vi "Append Inspection Waypoint.vi"(0 "Waypoint Array In":T1[](array[typedef]), 5 "Lat":sgl, 7 "Lon":sgl, 9 "Altitude (m)":sgl, 11 "Error In":errorcluster, 12 "Inspection altitude (m)":sgl=10.0, 13 "Capture Photo":bool) -> (4 "appended array":T1[](array[typedef]), 15 "Error Out":errorcluster)   [LabVIEW 2014]
uses:
  Controls/Mission Planning Controls/MAVLINK Mission Item.ctl
  Controls/MAVLINK Mav Frame.ctl
  Commands/Mission Planning/MISSION_ITEM SubVI/MISSION_ITEM Loiter (Time).vi
  Commands/Mission Planning/MISSION_ITEM SubVI/MISSION_ITEM Condition YAW.vi
  Commands/Mission Planning/MISSION_ITEM SubVI/MISSION_ITEM Take Photo.vi
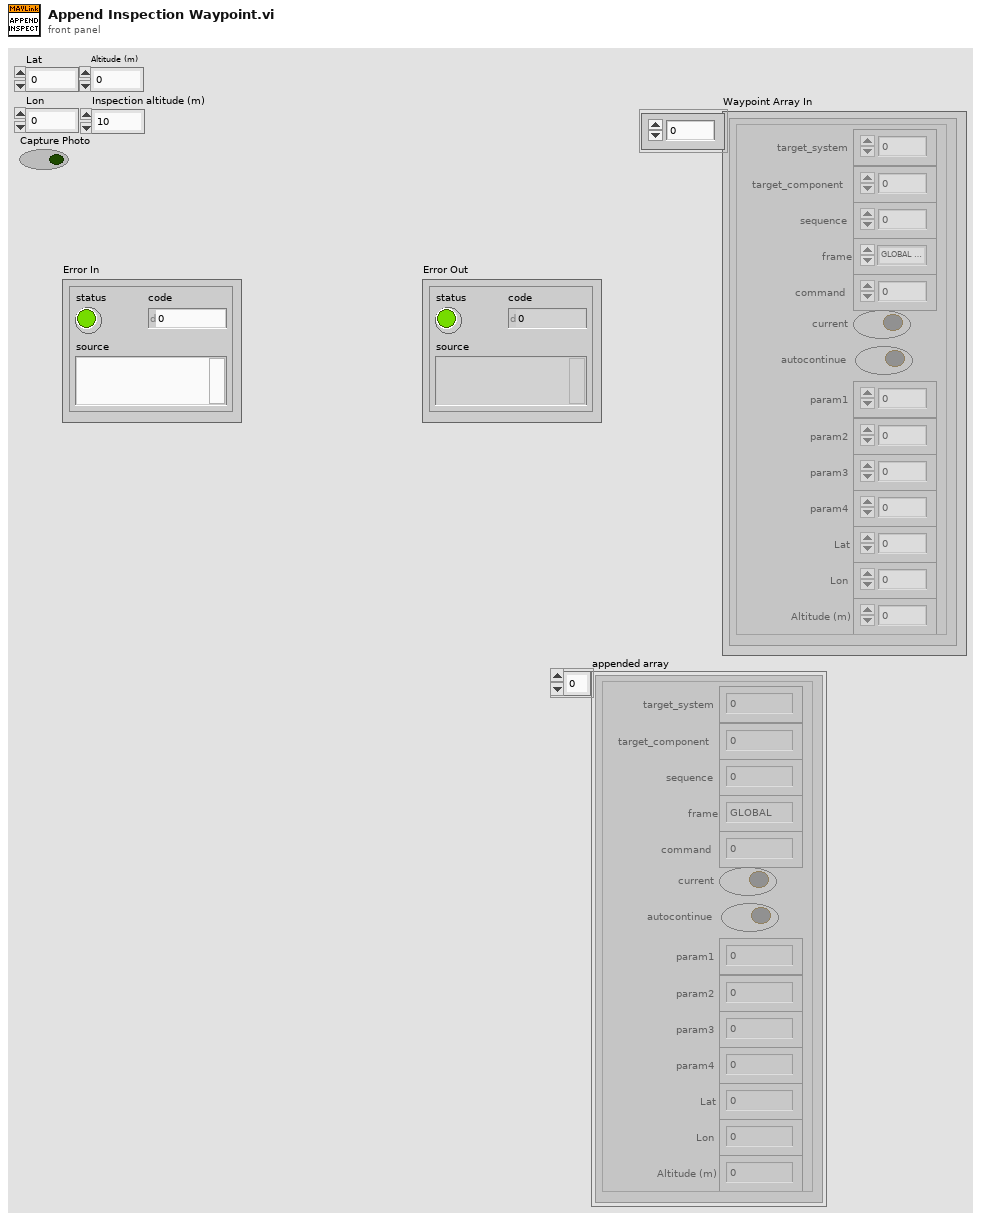
[diagram p1: front panel]
types:
  T1 = typedef "MAVLINK Mission Item.ctl" = cluster{"target_system":u8, "target_component":u8, "sequence":u16, "frame":T2, "command":u16, "current":bool, "autocontinue":bool, "param1":sgl, "param2":sgl, "param3":sgl, "param4":sgl, "Lat":sgl, "Lon":sgl, "Altitude (m)":sgl}
  T2 = typedef "MAVLINK Mav Frame.ctl" = enum8{"GLOBAL", "LOCAL NED", "MISSION", "GLOBAL RELATIVE ALT", "LOCAL ENU", "GLOBAL INT", "GLOBAL RELATIVE ALT INT", "LOCAL OFFSET NED", "BODY NED", "BODY OFFSET NED", "GLOBAL TERRAIN ALT", "GLOBAL TERRAIN ALT INT"}
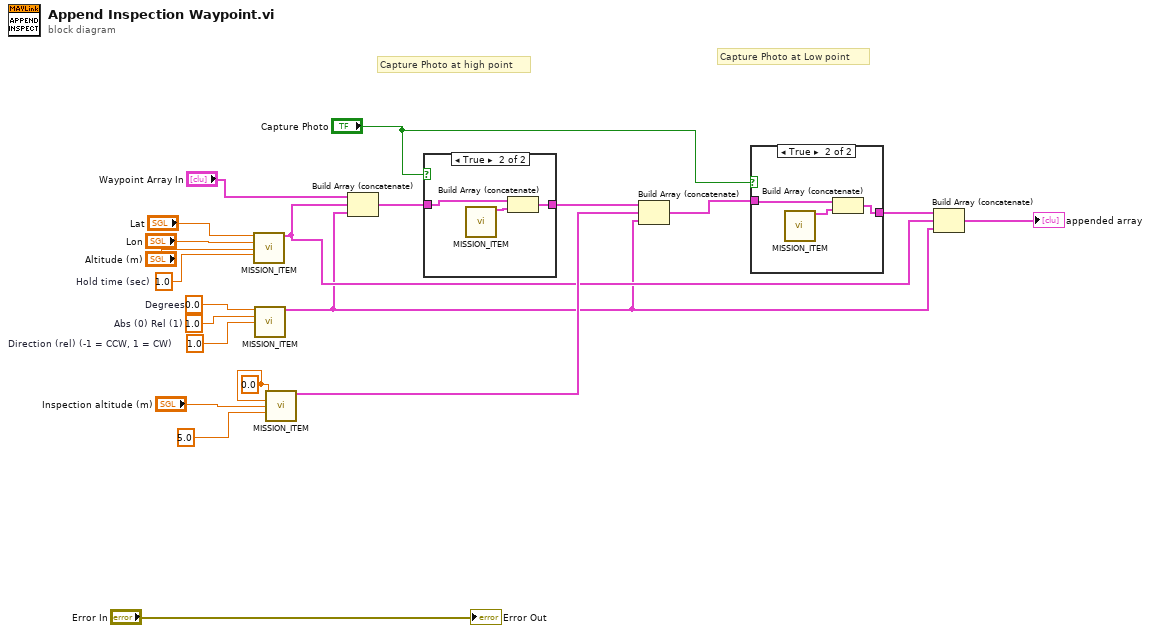
[diagram p0: block diagram]
diagram:
  w11 = sgl 1.0  # Direction (rel) (-1 = CCW, 1 = CW)
  w12 = sgl 1.0  # Abs (0) Rel (1)
  w13 = sgl 0.0  # Degrees
  w15 = sgl 0.0 ("Lat")
  w18 = sgl 1.0  # Hold time (sec)
  # "Capture Photo at Low point"
  # "Capture Photo at high point"
  n1 = call-poly "MISSION_ITEM.vi"("Lat"="Lat", "Lon"="Lon", "Altitude (m)"="Altitude (m)", "Loiter time (sec)"=w18) -> ("Mission Item"=w3:T1)  [unwired: 11 in]
  n2 = call-poly "MISSION_ITEM.vi"("Degrees"=w13, "Abs (0) Rel (1)"=w12, "Direction (rel) (-1 = CCW, 1 = CW)"=w11) -> ("Mission Item"=w2:T1)  [unwired: 12 in]
  n3 = call-poly "MISSION_ITEM.vi"("Lat"=w15, "Lon"=w15, "Altitude (m)"="Inspection altitude (m)", "Loiter time (sec)"=sgl 5.0) -> ("Mission Item"=w7:T1)  [unwired: 11 in]
  n4 = Build Array (concatenate)("Waypoint Array In", w3, w2) -> (w9:T1[])
  n5 = case shown="True" "Capture Photo" {
    tunnel: w9 -> [w22 w25]
    tunnel: [w22 w23] -> w8
    frame False {
    }
    frame True {
      n6 = call-poly "MISSION_ITEM.vi"() -> ("Mission Item"=w24:T1)  [unwired: 15 in]
      n7 = Build Array (concatenate)(w25, w24) -> (w23:T1[])
    }
  }
  n8 = Build Array (concatenate)(w8, w7, w2) -> (w6:T1[])
  n9 = case shown="True" "Capture Photo" {
    tunnel: w6 -> [w26 w29]
    tunnel: [w26 w27] -> w4
    frame False {
    }
    frame True {
      n10 = call-poly "MISSION_ITEM.vi"() -> ("Mission Item"=w28:T1)  [unwired: 15 in]
      n11 = Build Array (concatenate)(w29, w28) -> (w27:T1[])
    }
  }
  n12 = Build Array (concatenate)(w4, w3, w2) -> (→"appended array":T1[])
  "Error Out" <- "Error In"
